vi "Peregrine_eeprom_write.vi"(0 "Handle in":refnum<visa-resource-name>, 2 "Address":u8, 5 "eeprom address":u32, 9 "Value to be write":u32, 11 "error":errorcluster) -> (4 "Handle out":refnum<visa-resource-name>, 6 "Key response":u32, 8 "Value response":u32, 15 "error out":errorcluster)   [LabVIEW 2019]
panel:
  out "unsigned byte array":u8[](array[numeric])
  out "length 2":i32
  out "length":i32
  out "Command":i32
  out "Address response":u8
  # "Inputs"
  # "Response message"
  # "Output"
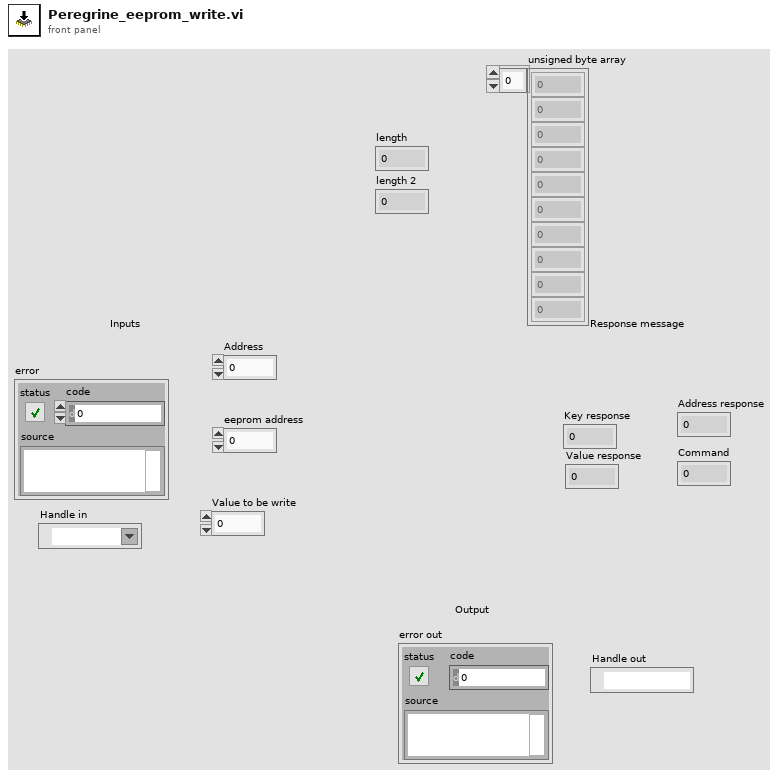
[diagram p1: front panel]
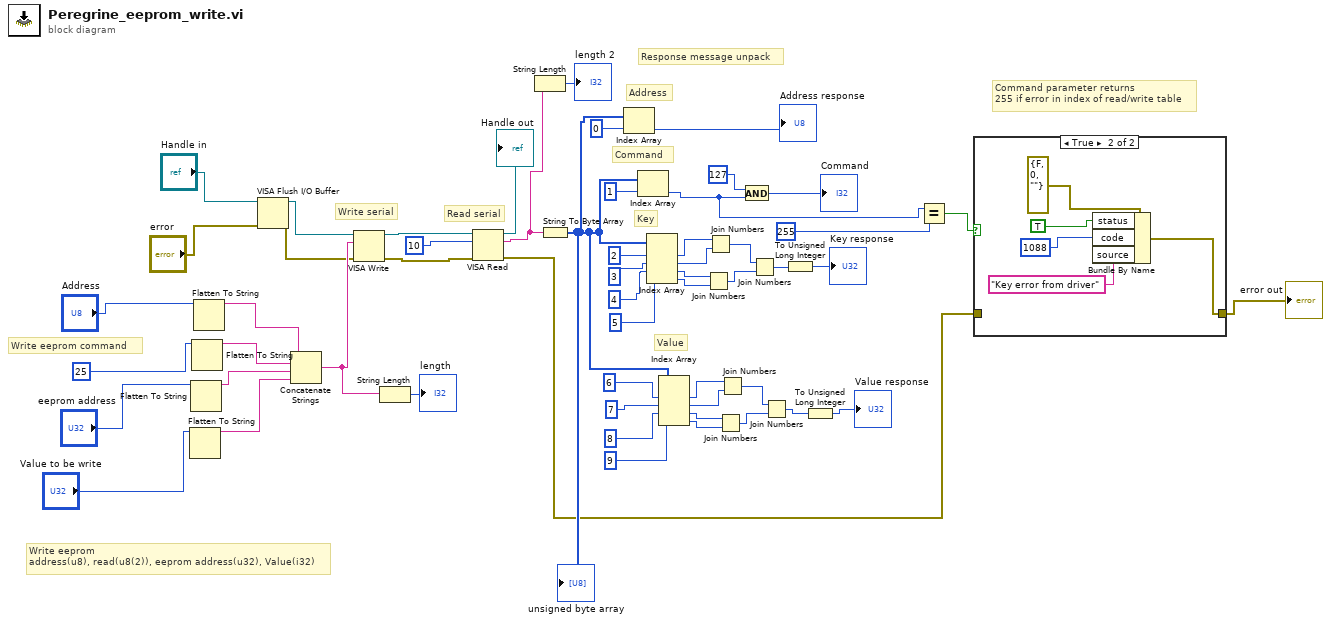
[diagram p0: block diagram]
diagram:
  # "Command parameter returns\n255 if error in index of read/write table"
  # "Value"
  # "Response message unpack"
  # "Write eeprom command"
  # "Command"
  # "Address"
  # "Key"
  # "Read serial"
  # "Write serial"
  # "Write eeprom\naddress(u8), read(u8(2)), eeprom address(u32), Value(i32)"
  n1 = Flatten To String(anything="Value to be write") -> (data string=w32:string)  [unwired: 3 in, 2 out]
  n2 = Flatten To String(anything="eeprom address") -> (data string=w33:string)  [unwired: 3 in, 2 out]
  n3 = Flatten To String(anything=u8 25) -> (data string=w12:string)  [unwired: 3 in, 2 out]
  n4 = Flatten To String(anything="Address") -> (data string=w35:string)  [unwired: 3 in, 2 out]
  n5 = VISA Flush I/O Buffer(VISA resource name="Handle in", error in (no error)="error") -> (VISA resource name out=w2:refnum<visa-resource-name>, error out=w1:errorcluster)  [unwired: 1 in]
  n6 = Concatenate Strings(w35, w12, w33, w32) -> (w8:string)
  n7 = VISA Write(VISA resource name=w2, write buffer=w8, error in (no error)=w1) -> (VISA resource name out=w55:refnum<visa-resource-name>, error out=w37:errorcluster)  [unwired: 1 out]
  n8 = String Length(string=w8) -> (length=→"length":i32)
  n9 = VISA Read(VISA resource name=w55, byte count=10, error in (no error)=w37) -> (VISA resource name out=→"Handle out":refnum<visa-resource-name>, read buffer=w6:string, error out=w14:errorcluster)  [unwired: 1 out]
  n10 = String Length(string=w6) -> (length=→"length 2":i32)
  n11 = String To Byte Array(string=w6) -> (unsigned byte array=w23:u8[])
  "unsigned byte array" <- w23
  n12 = Index Array(array=w23, index=0) -> (element=→"Address response":u8)
  n13 = Index Array(array=w23, index=1) -> (element=w17:u8)
  n14 = Index Array(array=w23, index #1=2, index #2=3, index #3=4, index #4=5) -> (element #1=w47:u8, element #2=w46:u8, element #3=w45:u8, element #4=w44:u8)
  n15 = Index Array(array=w23, index #1=6, index #2=7, index #3=8, index #4=9) -> (element #1=w30:u8, element #2=w29:u8, element #3=w28:u8, element #4=w27:u8)
  n16 = Join Numbers(hi=w45, lo=w44) -> ((hi.lo)=w43:u16)
  n17 = Join Numbers(hi=w47, lo=w46) -> ((hi.lo)=w42:u16)
  n18 = Join Numbers(hi=w28, lo=w27) -> ((hi.lo)=w26:u16)
  n19 = Join Numbers(hi=w30, lo=w29) -> ((hi.lo)=w25:u16)
  n20 = And(x=127, y=w17) -> (x .and. y?=→"Command":i32)
  n21 = Join Numbers(hi=w42, lo=w43) -> ((hi.lo)=w19:u32)
  n22 = Join Numbers(hi=w25, lo=w26) -> ((hi.lo)=w10:u32)
  n23 = To Unsigned Long Integer(number=w19) -> (unsigned 32bit integer=→"Key response":u32)
  n24 = To Unsigned Long Integer(number=w10) -> (unsigned 32bit integer=→"Value response":u32)
  n25 = Equal?(x=w17, y=255) -> (x = y?=w15:bool)
  n26 = case shown="True" w15 {
    tunnel: w14 -> [w56 _]
    tunnel: [w56 w58] -> w13
    frame False {
    }
    frame True {
      n27 = Bundle By Name(cluster=errorcluster {"status"=FALSE, "code"=0, "source"=""} ("error constant"), "status"=TRUE, "code"=1088, "source"="Key error from driver") -> (w58:errorcluster)
    }
  }
  "error out" <- w13
